vi "load_execute.vi"(4 "token cluster in":T1, 6 "timeout (ms)":i32=10000, 7 "IP address":string, 8 "error in (no error)":errorcluster, 9 "Load action":string(combo)="LOAD_ACTION_OFF", 10 "Load number":u8=1 min=1 max=24 step=1, 11 "client handle":T2) -> (0 "error out":errorcluster, 1 "token cluster":T1, 3 "client handle out":T2)   [LabVIEW 2018]
uses:
  <vilib>/httpClient/ClientHandle.ctl
  <vilib>/httpClient/LabVIEWHTTPClient.lvlib
panel:
  out "return code":i32
  out "standard error":string
  out "curl request":string
  out "response (JSON)":string
  out "headers":string
  out "status code":string
  out "msg":string
  out "reponse":string
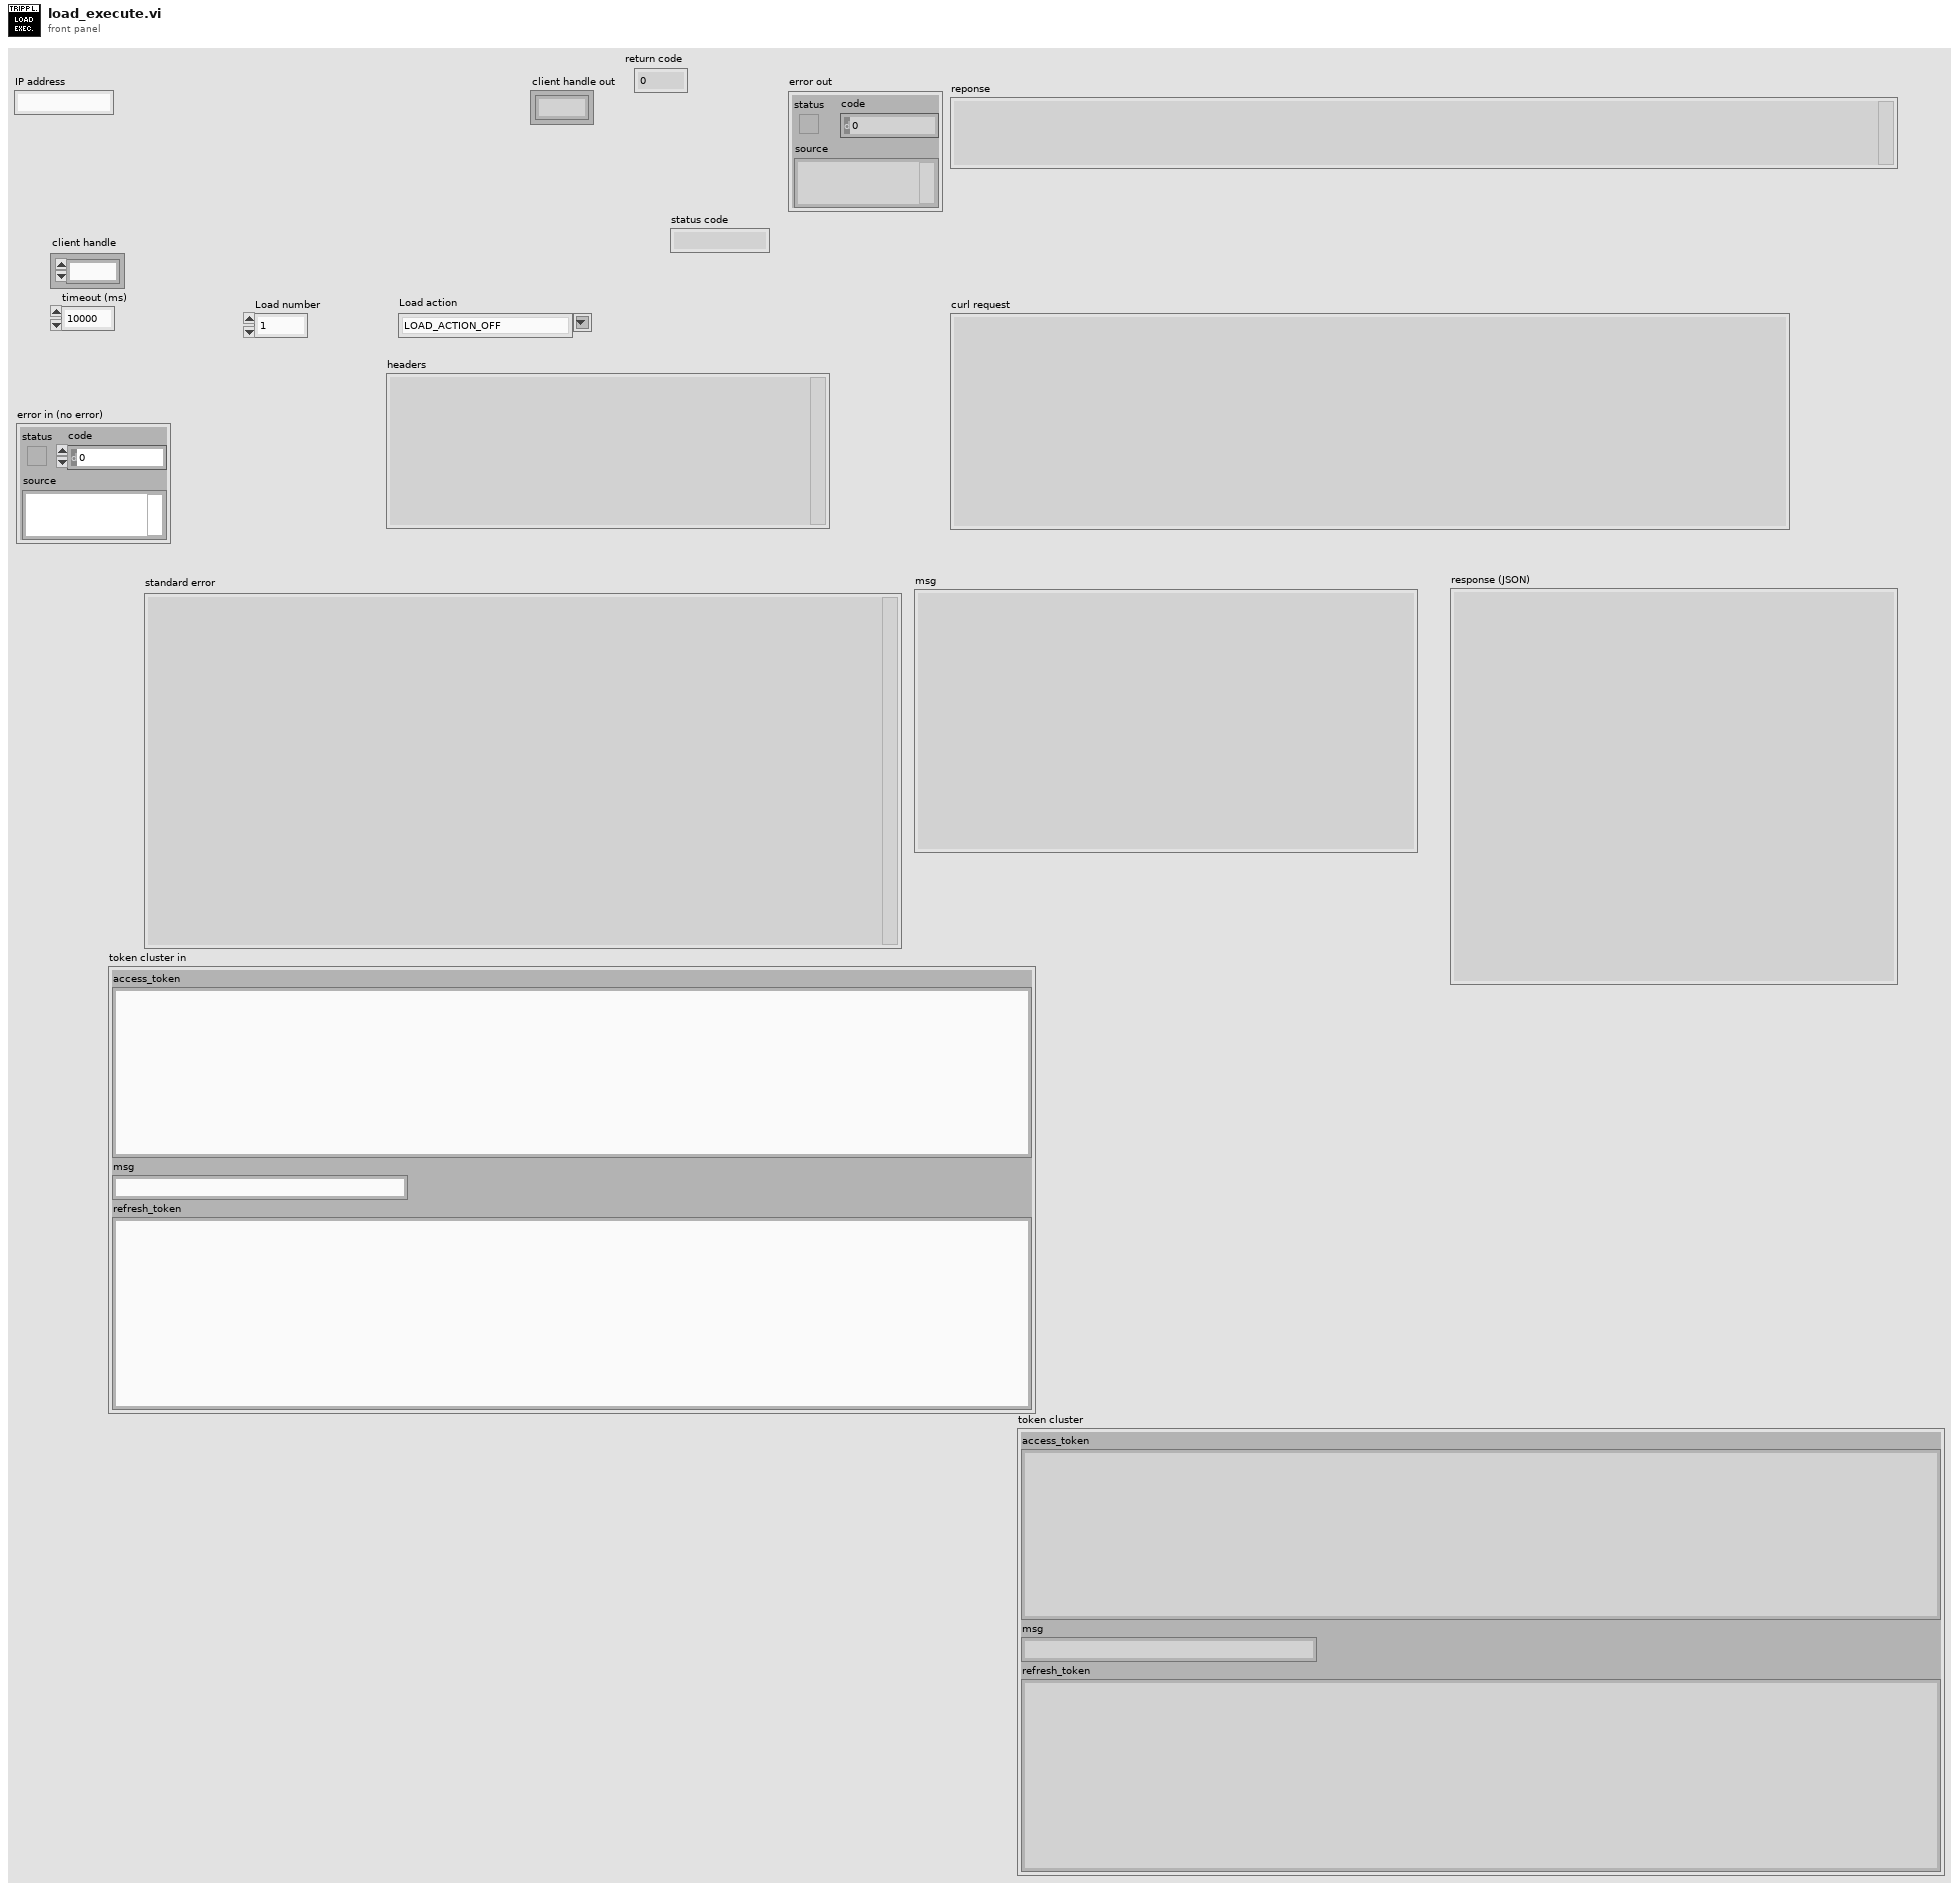
[diagram p1: front panel]
types:
  T1 = cluster{"access_token":string, "msg":string, "refresh_token":string}
  T2 = typedef "LabVIEWHTTPClient.lvlib/ClientHandle.ctl" = refnum<k1>
  T3 = cluster{"data":cluster{"type":string, "attributes":cluster{"device_id":i32, "load_action":string}}}
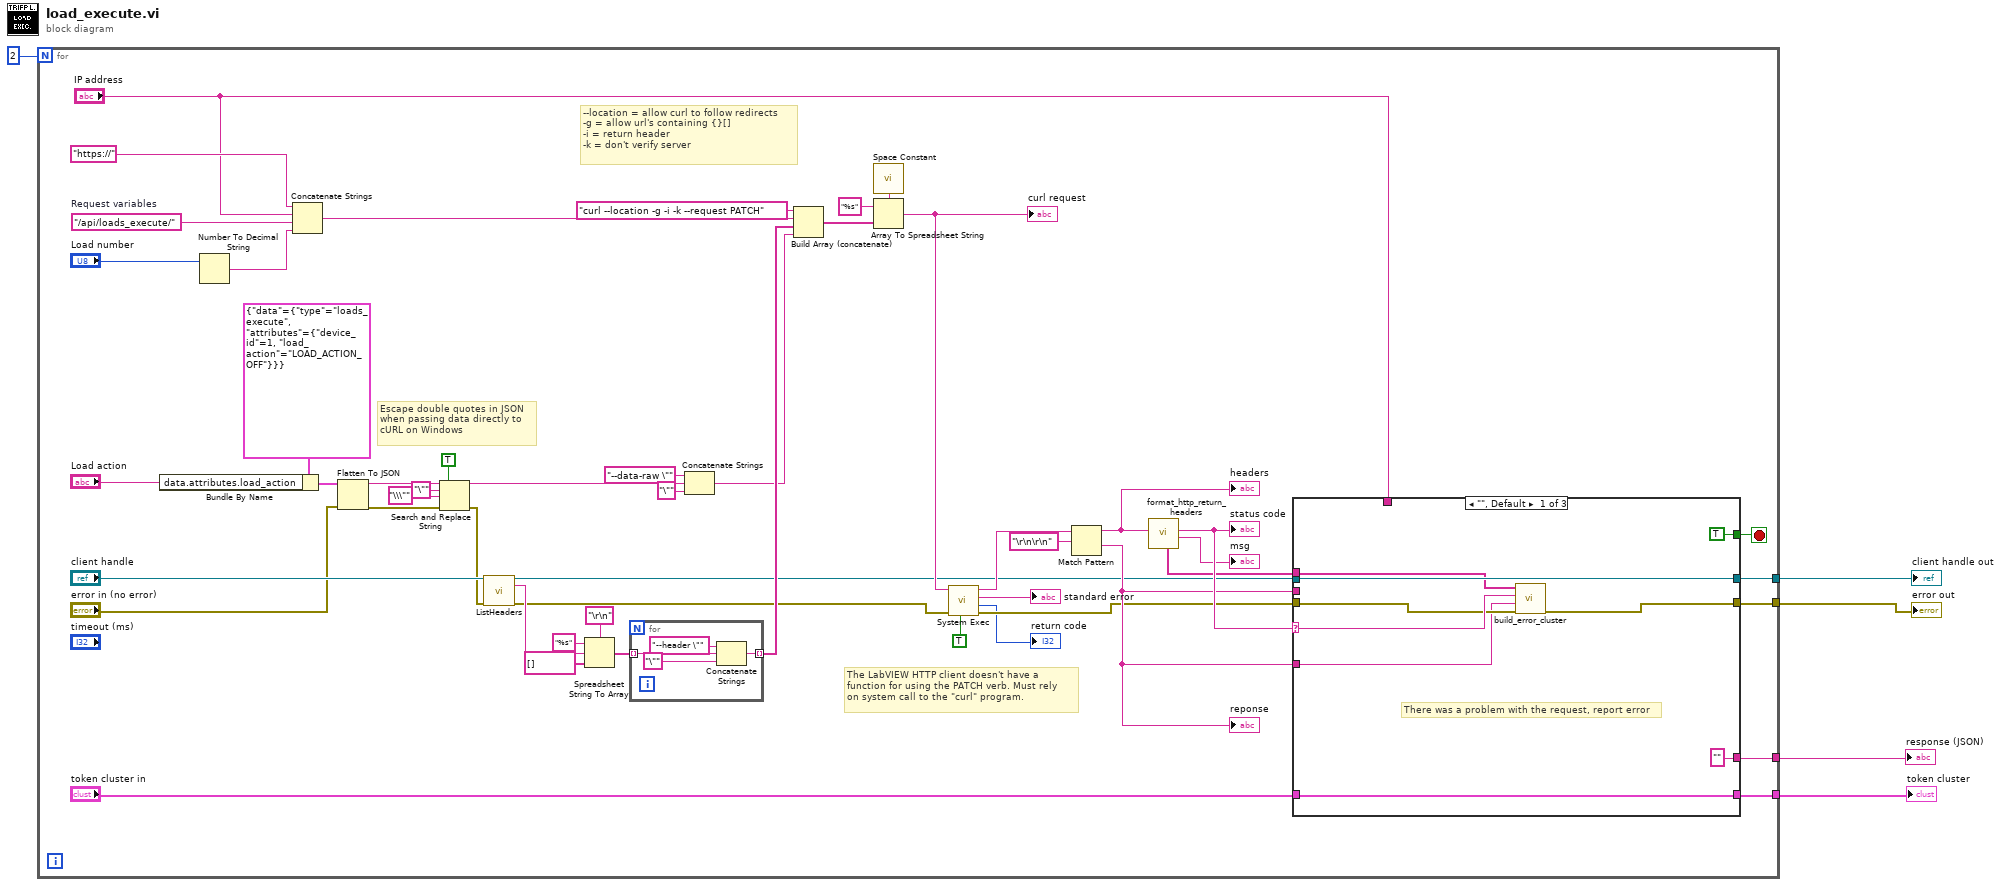
[diagram p0: block diagram]
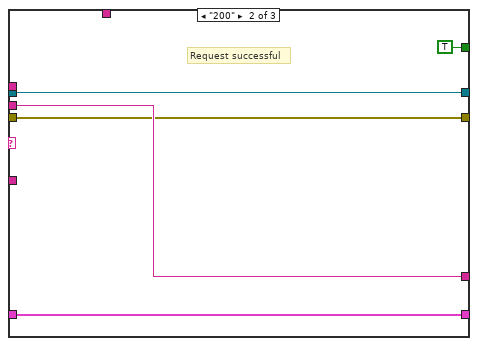
[diagram p2: hidden frame]
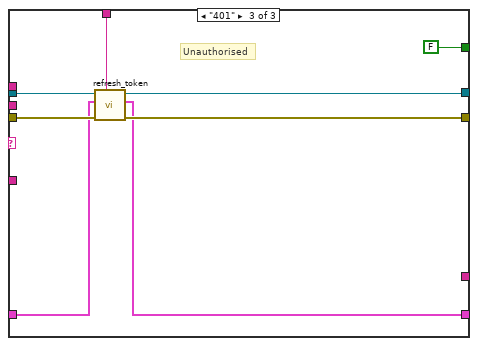
[diagram p3: hidden frame]
diagram:
  n1 = for {
    N: 2 -> [_]
    tunnel: [w54] -> w5
    tunnel: [w53] -> w4
    tunnel: [w49] -> w3
    tunnel: [w7] -> w1
    stop <- w6 stop-if-true
    w56 = "/api/loads_execute/"  # Request variables
    # "Escape double quotes in JSON\nwhen passing data directly to\ncURL on Windows"
    # "--location = allow curl to follow redirects \n-g = allow url's containing {}[]\n-i = return header\n-k = don't verify server"
    # "The LabVIEW HTTP client doesn't have a \nfunction for using the PATCH verb. Must rely\non system call to the \"curl\" program."
    n2 = Bundle By Name(cluster=T3 {"data"={"type"="loads_execute", "attributes"={"device_id"=1, "load_action"="LOAD_ACTION_OFF"}}}, "data.attributes.load_action"="Load action") -> (w26:T3)
    n3 = Number To Decimal String(number="Load number") -> (decimal integer string=w47:string)  [unwired: 1 in]
    n4 = Concatenate Strings("https://", "IP address", w56, w47) -> (w35:string)
    n5 = Flatten To JSON(anything=w26, error in (no error)="error in (no error)") -> (JSON string=w17:string, 11:w11:errorcluster)  [unwired: 1 in]
    n6 = Search and Replace String(replace all?=TRUE ("replace all? (F)"), input string=w17, search string="\"", replace string="\\\"" ("replace string (\"\")"), error in=w11) -> (result string=w14:string, error out=w10:errorcluster)  [unwired: 3 in, 2 out]
    n7 = call <vilib>:"ListHeaders.vi"("client handle"="client handle", "error in (no error)"=w10) -> ("client handle out"=w20:T2, "headers"=w34:string, "error out"=w12:errorcluster)  [unwired: 11 in]
    n8 = Spreadsheet String To Array(delimiter (Tab)="\r\n", format string="%s", spreadsheet string=w34, array type (2D Dbl)=string[] []) -> (array=w30:string[])
    n9 = for {
      tunnel: w30 -> [w57] mode=indexing
      tunnel: [w58] -> w29 mode=indexing
      n10 = Concatenate Strings("--header \"" ("string"), w57, "\"" ("string")) -> (w58:string)
    }
    n11 = Concatenate Strings("--data-raw \"" ("string"), w14, "\"" ("string")) -> (w23:string)
    n12 = Build Array (concatenate)("curl --location -g -i -k --request PATCH", w35, w29, w23) -> (w42:string[])
    n13 = call <vilib>:"Space Constant.vi"() -> ("String"=w45:string)
    n14 = Array To Spreadsheet String(delimiter (Tab)=w45, array=w42, 3:"%s" ("format string")) -> (spreadsheet string=w21:string)
    "curl request" <- w21
    n15 = call <vilib>:"System Exec.vi"("run minimized? (F)"=TRUE, "error in (no error)"=w12, "command line"=w21) -> ("error out"=w36:errorcluster, "return code"=→"return code":i32, "standard error"=→"standard error":string, "standard output"=w40:string)  [unwired: 5 in]
    n16 = Match Pattern(string=w40, regular expression="\r\n\r\n") -> (before substring=w38:string, after substring=w37:string)  [unwired: 1 in, 2 out]
    "reponse" <- w37
    "headers" <- w38
    n17 = call "format_http_return_headers.vi"("headers in"=w38) -> ("msg"=→"msg":string, "status code"=w52:string, "headers array"=w50:string[])  [unwired: 8 in]
    "status code" <- w52
    n18 = case shown="\"\", Default" w52 {
      selector: w52 -> [w68 _ _]
      tunnel: w36 -> [w66 w72 w82]
      tunnel: w37 -> [_ w74 _]
      tunnel: w20 -> [w69 w73 w78]
      tunnel: [w65 w72 w81] -> w54
      tunnel: [w69 w73 w79] -> w53
      tunnel: ["" ("body") w74 _] -> w49
      tunnel: w50 -> [w67 _ _]
      tunnel: w37 -> [w63 _ _]
      tunnel: "IP address" -> [_ _ w80]
      tunnel: "token cluster in" -> [w61 w70 w77]
      tunnel: [w61 w70 w76] -> w7
      tunnel: [TRUE TRUE FALSE] -> w6
      frame "", Default {
        # "There was a problem with the request, report error"
        n19 = call "build_error_cluster.vi"("error in (no error)"=w66, "error msg (JSON)"=w63, "status code"=w68, "headers array"=w67) -> ("error out"=w65:errorcluster)  [unwired: 7 in]
      }
      frame "200" {
        # "Request successful"
      }
      frame "401" {
        # "Unauthorised"
        n20 = call "refresh_token.vi"("IP address"=w80, "error in (no error)"=w82, "token cluster in"=w77, "client handle"=w78) -> ("error out"=w81:errorcluster, "token cluster"=w76:T1, "client handle out"=w79:T2)  [unwired: 5 in]
      }
    }
  }
  "error out" <- w5
  "client handle out" <- w4
  "response (JSON)" <- w3
  "token cluster" <- w1
